vi "FTW-File-UserDirectories.vi"(0 "Publisher (Organization)":string, 5 "Application (Product Name)":string) -> (4 "User Documents Dir":path, 6 "User Application Data Dir":path, 8 "User Preferences Dir":path, 10 "User Desktop":path)   [LabVIEW 2012]
panel:
  # "Inputs"
  # "Outputs"
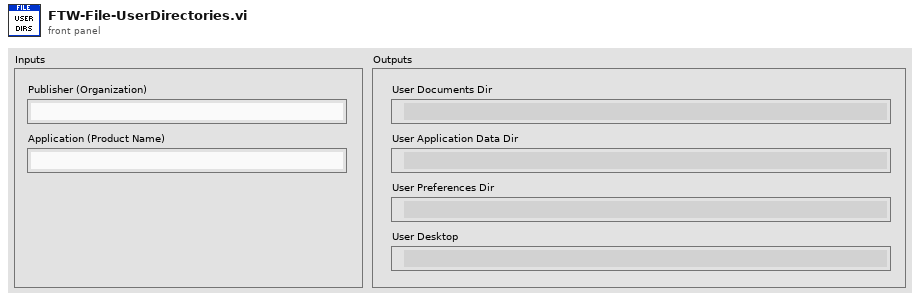
[diagram p1: front panel]
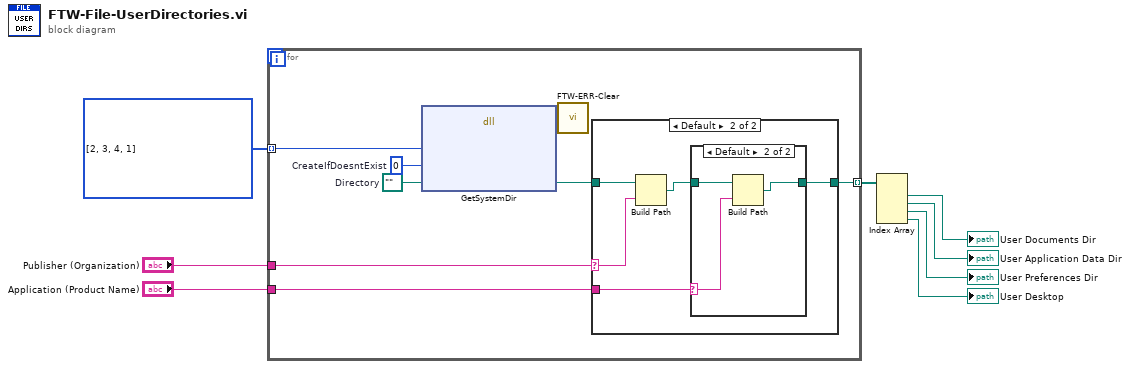
[diagram p0: block diagram]
diagram:
  w8 = i32[] [2, 3, 4, 1] items=["User Home"=0, "User Desktop"=1, "User Documents"=2, "User Application Data"=3, "User Preferences"=4, "User Temporary"=5, "Public Documents"=6, "Public Application Data"=7, "Public Preferences"=8, "Public Cache"=13, "System Core Libraries"=9, "System Installed Libraries"=10, "Application Files"=11, "Boot Volume Root"=12]
  n1 = for {
    tunnel: w8 -> [w13] mode=indexing
    tunnel: "Application (Product Name)" -> [w16]
    tunnel: [w15] -> w6 mode=indexing
    tunnel: "Publisher (Organization)" -> [w14]
    w11 = path ""  # Directory
    w12 = 0  # CreateIfDoesntExist
    n2 = dll-call lib="LabVIEW" fn="GetSystemDir"("System Directory Enum"=w13, "Create If Doesnt Exist"=w12, "Directory"=w11) -> (error out=w9:errorcluster, "Directory"=w10:path)  [unwired: 4 in, 3 out]
    n3 = call "FTW-ERR-Clear.vi"("error to snuff"=w9) -> ()  [unwired: 1 out]
    n4 = case shown="Default" w14 {
      selector: w14 -> [_ w18]
      tunnel: w10 -> [w17 w22]
      tunnel: w16 -> [_ w20]
      tunnel: [w17 w19] -> w15
      frame "" {
      }
      frame Default {
        n5 = Build Path(base path=w22, name or relative path=w18) -> (appended path=w21:path)
        n6 = case shown="Default" w20 {
          selector: w20 -> [_ w24]
          tunnel: w21 -> [w23 w26]
          tunnel: [w23 w25] -> w19
          frame "" {
          }
          frame Default {
            n7 = Build Path(base path=w26, name or relative path=w24) -> (appended path=w25:path)
          }
        }
      }
    }
  }
  n8 = Index Array(array=w6) -> (element #1=→"User Documents Dir":path, element #2=→"User Application Data Dir":path, element #3=→"User Preferences Dir":path, element #4=→"User Desktop":path)  [unwired: 4 in]
